vi "Initialize.vi"(0 "NSIS_Installer in":refnum<class "NSIS Installer.lvclass">) -> (4 "NSIS_Installer out":refnum<class "NSIS Installer.lvclass">)   [LabVIEW 2017, in "CL_G3_VIComponentBuilder.lvlib" / "NSIS Installer.lvclass"]
doc: "Responsible for determining the Unique Name, Product Name, and Export's Build Specification file."
uses:
  NSIS Installer.lvclass
  C:/Tool Chain Support/Software Module Builder/Source/Exports/Exports/Export.lvclass
  Exports/Export.lvclass/Export.ctl
  Exports/Accessors/Write Export Operation Errors.vi
  Exports/Accessors/Read Export Operation Errors.vi
  Exports/Accessors/Read Export Build Specification.vi
  Exports/Accessors/Write Product Name.vi
  Exports/Accessors/Write unique Name.vi
  Compound Installer/Compound_Installer.lvclass
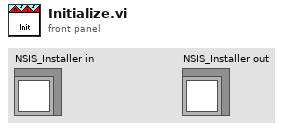
[diagram p1: front panel]
types:
  T1 = enum16{"open", "replace", "create", "open or create", "replace or create", "replace or create with confirmation"}
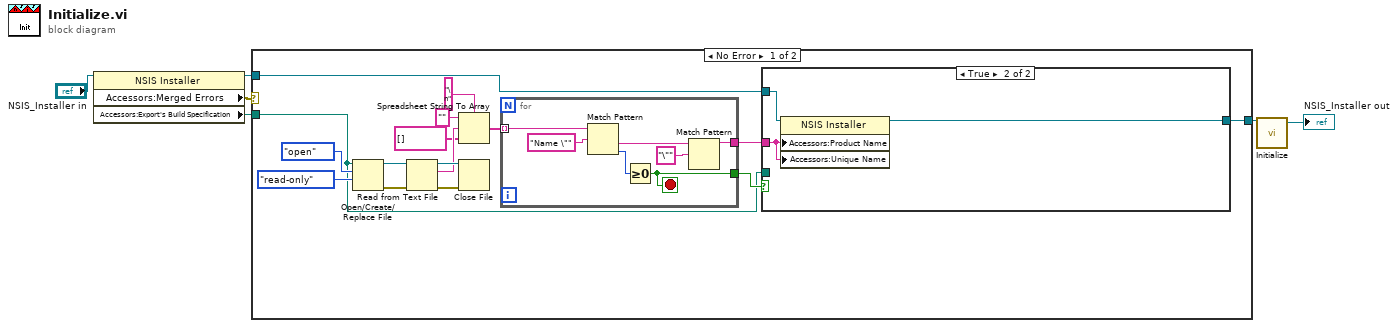
[diagram p0: block diagram]
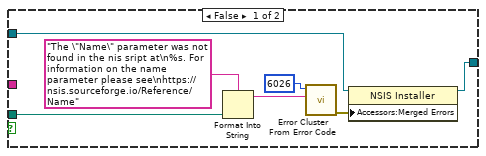
[diagram p2: hidden frame]
diagram:
  n1 = property class="NSIS Installer"(reference="NSIS_Installer in") -> (reference out=w5:refnum<class "NSIS Installer.lvclass">, "Accessors:Merged Errors"=w1:errorcluster, "Accessors:Export's Build Specification"=w3:path)  [unwired: 1 in, 1 out]
  n2 = case shown="No Error" w1 {
    tunnel: w5 -> [w16 w40]
    tunnel: [w12 w40] -> w4
    tunnel: w3 -> [w9 _]
    frame No Error {
      n3 = Open/Create/Replace File(file path (use dialog)=w9, operation (0:open)=T1."open", access (0:read/write)=enum16{"read/write", "read-only", "write-only"}."read-only") -> (refnum out=w21:refnum<file>, error out=w18:errorcluster)  [unwired: 3 in, 1 out]
      n4 = Read from Text File(file (use dialog)=w21, error in=w18) -> (refnum out=w22:refnum<file>, text=w15:string, error out=w17:errorcluster)  [unwired: 2 in, 1 out]
      n5 = Spreadsheet String To Array(delimiter (Tab)="\n", format string="", spreadsheet string=w15, array type (2D Dbl)=string[] []) -> (array=w13:string[])
      n6 = Close File(refnum=w22, error in=w17) -> ()  [unwired: 2 out]
      n7 = for {
        tunnel: w13 -> [w36] mode=indexing
        tunnel: [w34] -> w11
        tunnel: [w33] -> w10
        stop <- w33 stop-if-true
        n8 = Match Pattern(string=w36, regular expression="Name \"") -> (after substring=w39:string, offset past match=w35:i32)  [unwired: 1 in, 2 out]
        n9 = Greater Or Equal To 0?(x=w35) -> (x >= 0?=w33:bool)
        n10 = Match Pattern(string=w39, regular expression="\"") -> (before substring=w34:string)  [unwired: 1 in, 3 out]
      }
      n11 = case shown="True" w10 {
        tunnel: w16 -> [w29 w32]
        tunnel: [w28 w31] -> w12
        tunnel: w11 -> [_ w30]
        tunnel: w9 -> [w24 _]
        frame False {
          n12 = Format Into String(format string="The \"Name\" parameter was not found in the nis sript at\n%s. For information on the name parameter please see\nhttps://nsis.sourceforge.io/Reference/Name", w24) -> (resulting string=w27:string)  [unwired: 2 in, 1 out]
          n13 = call <vilib>:"Error Cluster From Error Code.vi"("error message (\"\")"=w27, "error code (0)"=6026) -> ("error out"=w23:errorcluster)  [unwired: 7 in]
          n14 = property class="NSIS Installer"(reference=w29, "Accessors:Merged Errors"=w23) -> (reference out=w28:refnum<class "NSIS Installer.lvclass">)  [unwired: 1 in, 1 out]
        }
        frame True {
          n15 = property class="NSIS Installer"(reference=w32, "Accessors:Product Name"=w30, "Accessors:Unique Name"=w30) -> (reference out=w31:refnum<class "NSIS Installer.lvclass">)  [unwired: 1 in, 1 out]
        }
      }
    }
    frame Error {
    }
  }
  n16 = call-parent "Initialize.vi"("NSIS_Installer in"=w4) -> ("NSIS_Installer out"=→"NSIS_Installer out":refnum<class "NSIS Installer.lvclass">)  [unwired: 14 in]
